vi "Configure Multi Eval Meas List Segment Carrier Component.vi"(0 "VISA resource name":refnum<visa-resource-name>, 1 "Center Frequency (1GHz)":dbl=1000000000.0 format="%#.9p", 2 "Physical Cell ID (0)":i32, 5 "Instance (1)":T3=1, 7 "Segment (1)":T2=1, 9 "Carrier Component (1)":T1=1, 11 "error in (no error)":errorcluster, 12 "Bandwidth (50 MHz)":i32(ring) items=["50 MHz", "100 MHz", "200 MHz", "400 MHz"], 13 "DMRS Type A Position (2)":i32=2) -> (4 "VISA resource name out":refnum<visa-resource-name>, 15 "error out":errorcluster)   [LabVIEW 2015, in "Rohde&Schwarz CMXP NR FR2 Measurement.lvlib"]
doc: "Configure the selected segment's carrier component.\n\nAttributes:\nRSCMXPNRFR2M_ATTR_MULTI_EVAL_MEASUREMENT_LIST_SEGMENT_CC_CENTER_FREQUENCY\nRSCMXPNRFR2M_ATTR_MULTI_EVAL_MEASUREMENT_LIST_SEGMENT_CC_BANDWIDTH\nRSCMXPNRFR2M_ATTR_MULTI_EVAL_MEASUREMENT_LIST_SEGMENT_CC_PHYSICAL_CELL_ID\nRSCMXPNRFR2M_ATTR_MULTI_EVAL_MEASUREMENT_LIST_SEGMENT_CC_DMRS_TYPE_A_POSITION\n\nRemote-control commands:\nCONFigure:NRMMw:MEAS<i>:LIST:SEGMent<no>[:CC<cc>]:FREQuency\nCONFigure:NRMMw:MEAS<i>:LIST:SEGMent<no>[:CC<cc>]:CBANdwidth\nCONFigure:NRMMw:MEAS<i>:LIST:SEGMent<no>[:CC<cc>]:PLCid\nCONFigure:NRMMw:MEAS<i>:LIST:SEGMent<no>[:CC<cc>]:TAPosition"
uses:
  <instrlib>/Rohde&Schwarz CMXP NR FR2 Measurement/Rohde&Schwarz CMXP NR FR2 Measurement.lvlib
  <instrlib>/Rohde&Schwarz CMXP NR FR2 Measurement/Private/_Instance.ctl
  <instrlib>/Rohde&Schwarz CMXP NR FR2 Measurement/Private/_Segment.ctl
  <instrlib>/Rohde&Schwarz CMXP NR FR2 Measurement/Private/_Carrier Component.ctl
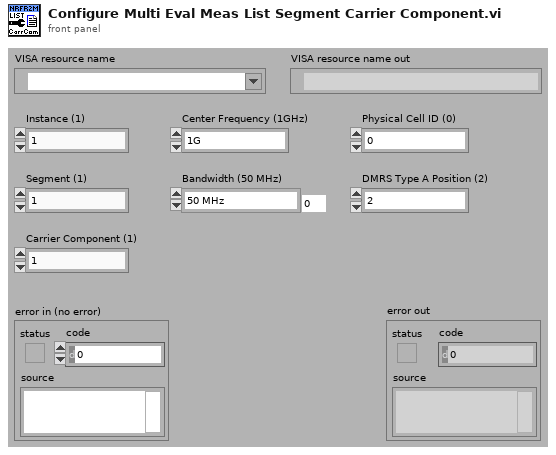
[diagram p1: front panel]
types:
  T1 = typedef "Rohde&Schwarz CMXP NR FR2 Measurement.lvlib/_Carrier Component.ctl" = i32
  T2 = typedef "Rohde&Schwarz CMXP NR FR2 Measurement.lvlib/_Segment.ctl" = i32
  T3 = typedef "Rohde&Schwarz CMXP NR FR2 Measurement.lvlib/_Instance.ctl" = i32
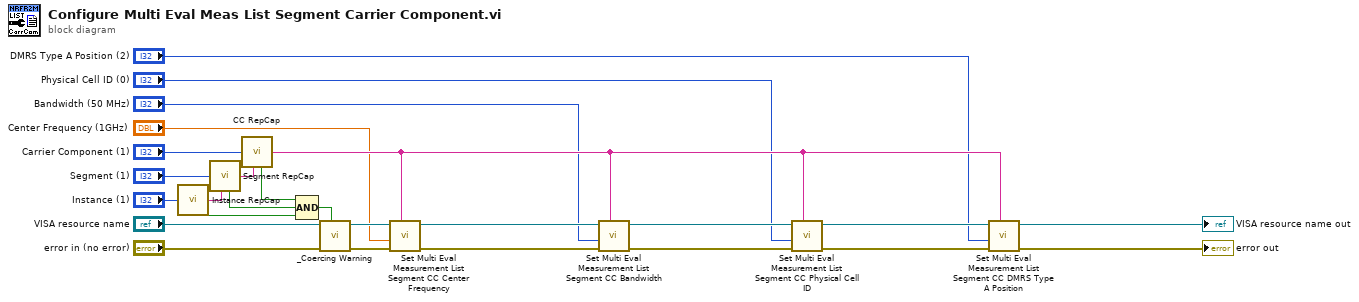
[diagram p0: block diagram]
diagram:
  n1 = call <instrlib>:"Instance RepCap.vi"("Instance In"="Instance (1)") -> ("In Range?"=w13:bool, "RepCap Identifier Out"=w5:string)  [unwired: 1 in]
  n2 = call <instrlib>:"Segment RepCap.vi"("Segment In"="Segment (1)", "RepCap String In (\"\")"=w5) -> ("In Range?"=w12:bool, "RepCap Identifier Out"=w11:string)
  n3 = call <instrlib>:"CC RepCap.vi"("CC In"="Carrier Component (1)", "RepCap String In (\"\")"=w11) -> ("In Range?"=w10:bool, "RepCap Identifier Out"=w7:string)
  n4 = Compound Arithmetic op=AND(w10, w12, w13) -> (w16:bool)
  n5 = call <instrlib>:"_Coercing Warning.vi"("In Range?"=w16, "error in (no error)"="error in (no error)", "VISA resource name"="VISA resource name") -> ("error out"=w8:errorcluster, "VISA resource name out"=w9:refnum<visa-resource-name>)  [unwired: 7 in]
  n6 = call "Set Multi Eval Measurement List Segment CC Center Frequency"("Repeated Capabilities"=w7, "error in (no error)"=w8, "Multi Eval Measurement List Segment CC Center Frequency (0.0)"="Center Frequency (1GHz)", "instrument handle"=w9) -> ("error out"=w25:errorcluster, "instrument handle out"=w26:refnum<visa-resource-name>)  [unwired: 6 in]
  n7 = call "Set Multi Eval Measurement List Segment CC Bandwidth"("Repeated Capabilities"=w7, "error in (no error)"=w25, "Multi Eval Measurement List Segment CC Bandwidth (0 - 50 MHz)"="Bandwidth (50 MHz)", "instrument handle"=w26) -> ("error out"=w23:errorcluster, "instrument handle out"=w24:refnum<visa-resource-name>)  [unwired: 6 in]
  n8 = call "Set Multi Eval Measurement List Segment CC Physical Cell ID"("Repeated Capabilities"=w7, "error in (no error)"=w23, "Multi Eval Measurement List Segment CC Physical Cell ID (0)"="Physical Cell ID (0)", "instrument handle"=w24) -> ("error out"=w19:errorcluster, "instrument handle out"=w20:refnum<visa-resource-name>)  [unwired: 6 in]
  n9 = call "Set Multi Eval Measurement List Segment CC DMRS Type A Position"("Repeated Capabilities"=w7, "error in (no error)"=w19, "Multi Eval Measurement List Segment CC DMRS Type A Position (0)"="DMRS Type A Position (2)", "instrument handle"=w20) -> ("error out"=→"error out":errorcluster, "instrument handle out"=→"VISA resource name out":refnum<visa-resource-name>)  [unwired: 6 in]
